vi "Error.vi"(8 "error in (no error)":errorcluster, 11 "Data":variant) -> (0 "error out":errorcluster)   [LabVIEW 2026, in "Sensor.lvlib"]
doc: "For named purposes"
uses:
  Sensor.lvlib
  Private Control/Queue Element.ctl
  Private Control/Module Action.ctl
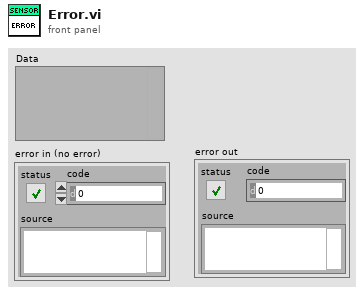
[diagram p1: front panel]
types:
  T1 = typedef "Sensor.lvlib/Queue Element.ctl" = cluster{"Module Action":T2, "Data":variant}
  T2 = typedef "Sensor.lvlib/Module Action.ctl" = enum16{"Init", "Error", "Exit"}
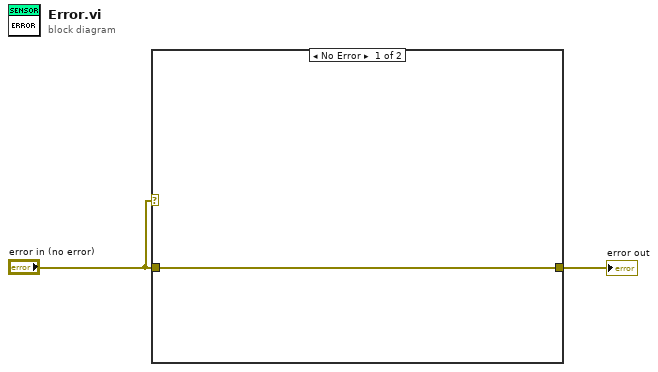
[diagram p0: block diagram]
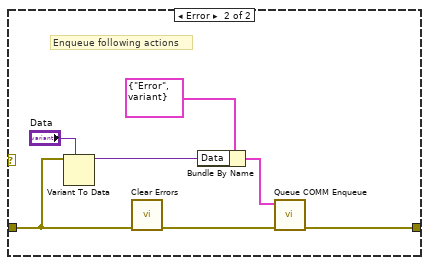
[diagram p2: hidden frame]
diagram:
  n1 = case shown="No Error" "error in (no error)" {
    tunnel: "error in (no error)" -> [w3 w5]
    tunnel: [w3 w8] -> w2
    frame No Error {
    }
    frame Error {
      # "Enqueue following actions"
      n2 = Variant To Data(type="Data", Variant=w5) -> (data=w4:variant)  [unwired: 1 in, 1 out]
      n3 = call <vilib>:"Clear Errors.vi"("error in (no error)"=w5) -> ("error out"=w7:errorcluster)  [unwired: 5 in, 1 out]
      n4 = Bundle By Name(cluster=T1 {"Module Action"=enum."Error", "Data"=variant} ("element"), "Data"=w4) -> (w9:T1)
      n5 = call "Queue COMM Enqueue.vi"("error in (no error)"=w7, "element"=w9) -> ("error out"=w8:errorcluster)  [unwired: 9 in]
    }
  }
  "error out" <- w2
